vi "Read.vi"(8 "error in":errorcluster, 11 "4-20mA Settings Input":T1) -> (0 "error out":errorcluster, 1 "Connection Error":bool, 2 "Read":dbl, 3 "4-20mA Settings Output":T1)   [LabVIEW 2018, in "Pressure Transmitter Library.lvlib"]
uses:
  Pressure Transmitter Library.lvlib
  <vilib>/DAQmx/read.llb/DAQmx Read (Analog DBL 1Chan 1Samp).vi
  Pressure Transmitter Device Settings.ctl
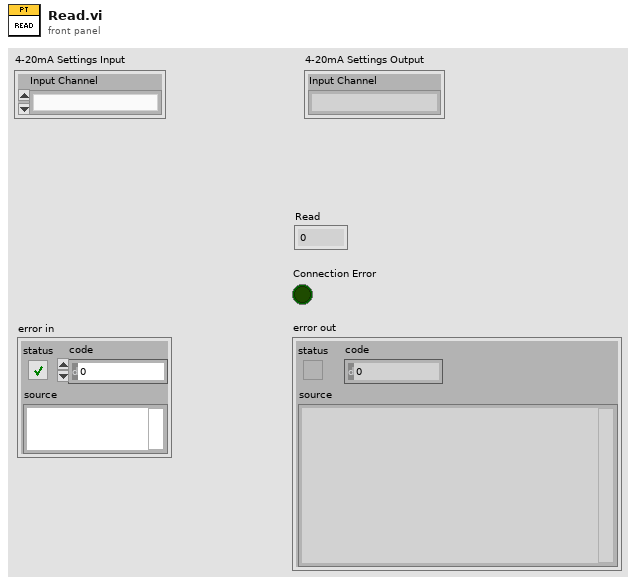
[diagram p1: front panel]
types:
  T1 = typedef "Pressure Transmitter Library.lvlib/Pressure Transmitter Device Settings.ctl" = cluster{"Input Channel ":enum16{""}}
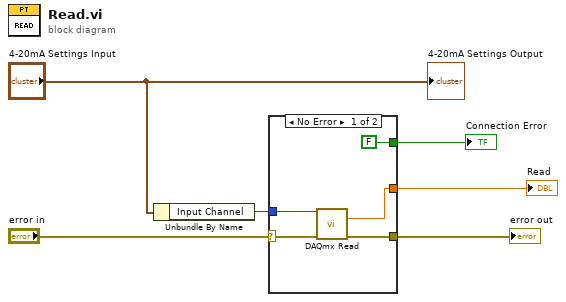
[diagram p0: block diagram]
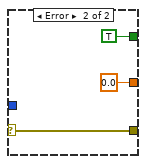
[diagram p2: hidden frame]
diagram:
  n1 = Unbundle By Name("4-20mA Settings Input") -> ("Input Channel"=w5:enum16{""})
  n2 = case shown="No Error" "error in" {
    selector: "error in" -> [w9 w13]
    tunnel: w5 -> [w11 _]
    tunnel: [w10 w13] -> w4
    tunnel: [FALSE ("Pump On?") TRUE ("Pump On?")] -> w1
    tunnel: [w8 0.0 ("data")] -> w2
    frame No Error {
      n3 = call-poly <vilib>:"DAQmx Read.vi"("task/channels in"=w11, "error in"=w9) -> ("data"=w8:dbl, "error out"=w10:errorcluster)  [unwired: 11 in, 1 out]
    }
    frame Error {
    }
  }
  "error out" <- w4
  "Connection Error" <- w1
  "Read" <- w2
  "4-20mA Settings Output" <- "4-20mA Settings Input"
